vi "余氯校准界面.vi"() -> ()   [LabVIEW 2016, in "斯坦道多参数.lvlib"]
panel:
  out "序列号":string caption="序列号："
  in  "余氯灵敏度校准":dbl=5.0 caption="余氯灵敏度校准：" format="%#.2f"
  in  "余氯零点校准":dbl caption="余氯零点校准：" format="%#.2f"
  in  "温度偏置":dbl=25.0 caption="温度偏置：" format="%#.2f"
  in  "氯偏置":dbl=25.0 caption="氯偏置：" format="%#.2f"
  in  "pH补偿值":dbl=25.0 caption="pH补偿值：" format="%#.2f"
  out "氯电压":dbl=25.0 caption="氯电压：" format="%#.2f mV"
  out "温度电压":dbl=25.0 caption="温度电压：" format="%#.2f mV"
  out "温度值":dbl=25.0 caption="温度值：" format="%#.2f"
  out "余氯值":dbl=25.0 caption="余氯值：" format="%#.2f"
  # "显示值<0.1时，用零点校准"
  # "显示值>0.1时，用灵敏度校准"
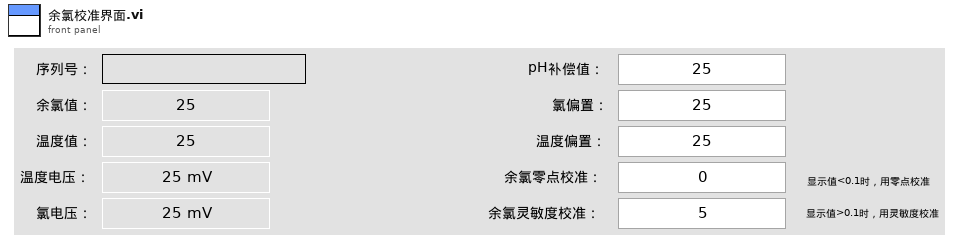
[diagram p1: front panel]
types:
  T1 = cluster{"余氯值":sgl, "温度值":sgl, "温度电压_mv":sgl, "氯电压_mv":dbl, "pH补偿值":dbl, "氯偏置":dbl, "温度偏置":dbl, "序列号":string}
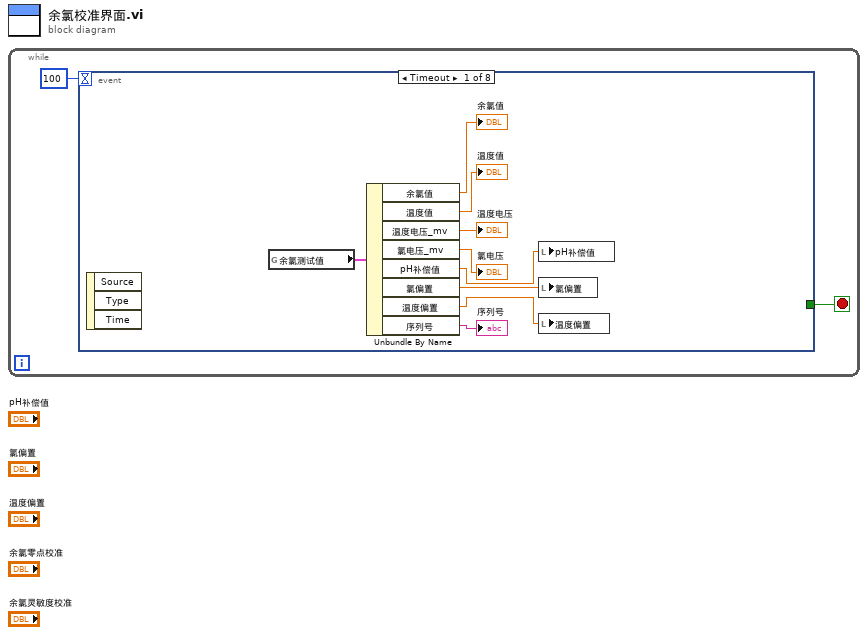
[diagram p0: block diagram]
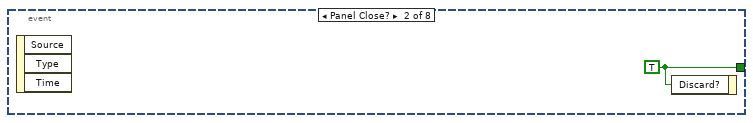
[diagram p2: hidden frame]
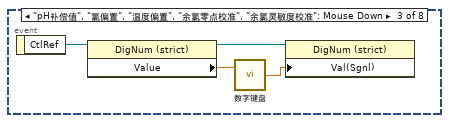
[diagram p3: hidden frame]
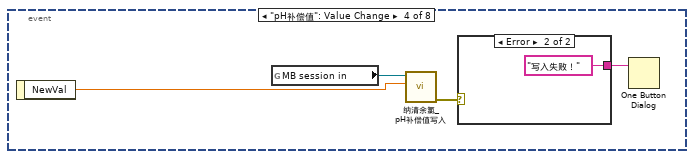
[diagram p4: hidden frame]
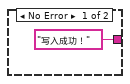
[diagram p5: hidden frame]
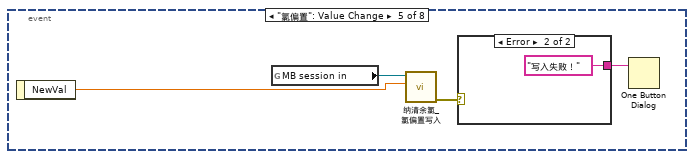
[diagram p6: hidden frame]
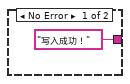
[diagram p7: hidden frame]
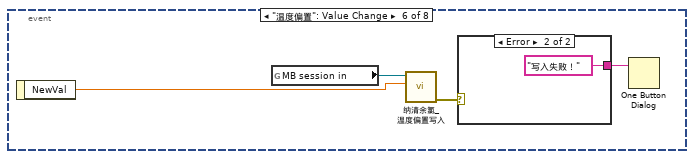
[diagram p8: hidden frame]
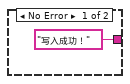
[diagram p9: hidden frame]
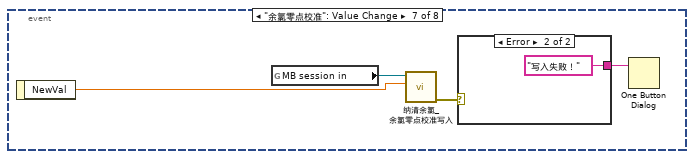
[diagram p10: hidden frame]
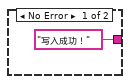
[diagram p11: hidden frame]
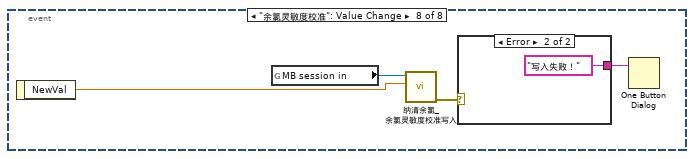
[diagram p12: hidden frame]
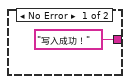
[diagram p13: hidden frame]
diagram:
  n1 = while {
    stop <- w1 stop-if-true
    n2 = event shown="[0] Timeout" {
      selector: _ -> [_ _ _ _ _ _ _ _]
      dyn-events: _ -> [_ _ _ _ _ _ _ _]
      timeout: 100 -> [_ _ _ _ _ _ _ _]
      tunnel: [_ w12 _ _ _ _ _ _] -> w1
      event Timeout {
        n3 = event-data() -> ()  [unwired: 1 in, 3 out]
        n4 = global read "纳清过程全局变量.vi" "余氯测试值"() -> (w11:T1)
        n5 = Unbundle By Name(w11) -> ("余氯值"=→"余氯值":sgl, "温度值"=→"温度值":sgl, "温度电压_mv"=→"温度电压":sgl, "氯电压_mv"=→"氯电压":dbl, "pH补偿值"=w6:dbl, "氯偏置"=w5:dbl, "温度偏置"=w4:dbl, "序列号"=→"序列号":string)
        n6 = local write "pH补偿值"(w6) -> ()
        n7 = local write "氯偏置"(w5) -> ()
        n8 = local write "温度偏置"(w4) -> ()
      }
      event Panel Close? {
        w12 = TRUE ("Discard?")
        n9 = event-data() -> ()  [unwired: 1 in, 3 out]
        n10 = event-data("Discard?"=w12) -> ()  [unwired: 1 in, 1 out]
      }
      event "pH补偿值", "氯偏置", "温度偏置", "余氯零点校准", "余氯灵敏度校准": Mouse Down {
        n11 = event-data() -> ("CtlRef"=w13:refnum<vi>)  [unwired: 1 in]
        n12 = property class="DigNum (strict)"(reference=w13) -> (reference out=w15:refnum<vi>, "Value"=w16:dbl)  [unwired: 1 in, 1 out]
        n13 = call "数字键盘.vi"("OldNumber"=w16) -> ("NewNumber"=w14:dbl)  [unwired: 1 in]
        n14 = property class="DigNum (strict)"(reference=w15, "Val(Sgnl)"=w14) -> ()  [unwired: 1 in, 2 out]
      }
      event "pH补偿值": Value Change {
        n15 = event-data() -> ("NewVal"=w18:dbl)  [unwired: 1 in]
        n16 = global read "多参数全局变量.vi" "MB session in"() -> (w19:refnum<class "MB_Master.lvclass">)
        n17 = call "纳清余氯_pH补偿值写入.vi"("数值"=w18, "MB session in"=w19) -> ("error out"=w17:errorcluster)  [unwired: 8 in, 1 out]
        n18 = case shown="Error" w17 {
          tunnel: ["写入成功！" "写入失败！"] -> w20
          frame No Error {
          }
          frame Error {
          }
        }
        n19 = One Button Dialog(message=w20) -> ()  [unwired: 1 in, 1 out]
      }
      event "氯偏置": Value Change {
        n20 = event-data() -> ("NewVal"=w24:dbl)  [unwired: 1 in]
        n21 = global read "多参数全局变量.vi" "MB session in"() -> (w25:refnum<class "MB_Master.lvclass">)
        n22 = call "纳清余氯_氯偏置写入.vi"("数值"=w24, "MB session in"=w25) -> ("error out"=w23:errorcluster)  [unwired: 8 in, 1 out]
        n23 = case shown="Error" w23 {
          tunnel: ["写入成功！" "写入失败！"] -> w26
          frame No Error {
          }
          frame Error {
          }
        }
        n24 = One Button Dialog(message=w26) -> ()  [unwired: 1 in, 1 out]
      }
      event "温度偏置": Value Change {
        n25 = event-data() -> ("NewVal"=w30:dbl)  [unwired: 1 in]
        n26 = global read "多参数全局变量.vi" "MB session in"() -> (w31:refnum<class "MB_Master.lvclass">)
        n27 = call "纳清余氯_温度偏置写入.vi"("数值"=w30, "MB session in"=w31) -> ("error out"=w29:errorcluster)  [unwired: 8 in, 1 out]
        n28 = case shown="Error" w29 {
          tunnel: ["写入成功！" "写入失败！"] -> w32
          frame No Error {
          }
          frame Error {
          }
        }
        n29 = One Button Dialog(message=w32) -> ()  [unwired: 1 in, 1 out]
      }
      event "余氯零点校准": Value Change {
        n30 = event-data() -> ("NewVal"=w36:dbl)  [unwired: 1 in]
        n31 = global read "多参数全局变量.vi" "MB session in"() -> (w37:refnum<class "MB_Master.lvclass">)
        n32 = call "纳清余氯_余氯零点校准写入.vi"("数值"=w36, "MB session in"=w37) -> ("error out"=w35:errorcluster)  [unwired: 8 in, 1 out]
        n33 = case shown="Error" w35 {
          tunnel: ["写入成功！" "写入失败！"] -> w38
          frame No Error {
          }
          frame Error {
          }
        }
        n34 = One Button Dialog(message=w38) -> ()  [unwired: 1 in, 1 out]
      }
      event "余氯灵敏度校准": Value Change {
        n35 = event-data() -> ("NewVal"=w42:dbl)  [unwired: 1 in]
        n36 = global read "多参数全局变量.vi" "MB session in"() -> (w43:refnum<class "MB_Master.lvclass">)
        n37 = call "纳清余氯_余氯灵敏度校准写入.vi"("数值"=w42, "MB session in"=w43) -> ("error out"=w41:errorcluster)  [unwired: 8 in, 1 out]
        n38 = case shown="Error" w41 {
          tunnel: ["写入成功！" "写入失败！"] -> w44
          frame No Error {
          }
          frame Error {
          }
        }
        n39 = One Button Dialog(message=w44) -> ()  [unwired: 1 in, 1 out]
      }
    }
  }
